vi "Events.vi"() -> ()   [LabVIEW 2019]
panel:
  out "Clock":string
  in  "Stop":bool
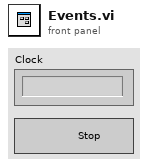
[diagram p1: front panel]
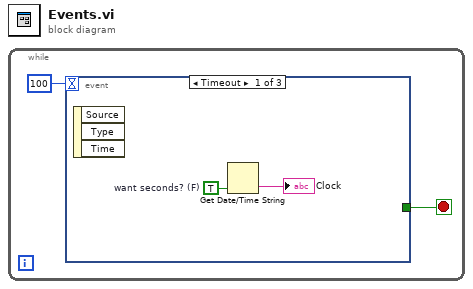
[diagram p0: block diagram]
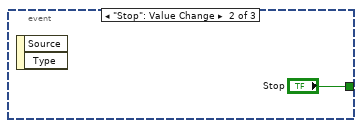
[diagram p2: hidden frame]
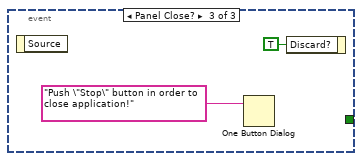
[diagram p3: hidden frame]
diagram:
  n1 = while {
    stop <- w1 stop-if-true
    n2 = event shown="[0] Timeout" {
      selector: _ -> [_ _ _]
      dyn-events: _ -> [_ _ _]
      timeout: 100 -> [_ _ _]
      tunnel: [_ "Stop" _] -> w1
      event Timeout {
        w4 = TRUE  # want seconds? (F)
        n3 = event-data() -> ()  [unwired: 1 in, 3 out]
        n4 = Get Date/Time String(want seconds? (F)=w4) -> (time string=→"Clock":string)  [unwired: 2 in, 1 out]
      }
      event "Stop": Value Change {
        n5 = event-data() -> ()  [unwired: 1 in, 2 out]
      }
      event Panel Close? {
        n6 = event-data() -> ()  [unwired: 1 in, 1 out]
        n7 = One Button Dialog(message="Push \"Stop\" button in order to close application!") -> ()  [unwired: 1 in, 1 out]
        n8 = event-data("Discard?"=TRUE) -> ()  [unwired: 1 in, 1 out]
      }
    }
  }
